vi "Run All Tests.vi"(8 "error in (no error)":errorcluster, 11 "Execution UI In":refnum<class "Execution UI V2.lvclass">) -> (0 "error out":errorcluster, 3 "Execution UI Out":refnum<class "Execution UI V2.lvclass">)   [LabVIEW 2020, in "Execution UI V2.lvclass"]
uses:
  Execution UI V2.lvclass
  Execution UI V2.lvclass/Execution UI V2.ctl
  Run/Runnable.lvclass
  Result Model/Result Model.lvclass
  TypeDefs/Execution State.ctl
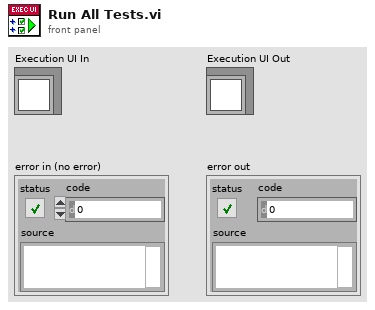
[diagram p1: front panel]
types:
  T1 = typedef "Execution UI V2.lvclass/Execution State.ctl" = enum16{"Idle", "Running"}
  T2 = typedef "Result.lvlib/Result.ctl" = cluster{"Name":string, "Message":string, "Description":string, "Status":T3, "Result Type":T4, "Execution Time":dbl}
  T3 = typedef "Result.lvlib/Status.ctl" = enum16{"", "Passed", "Failed", "Error", "Skipped", "Setup Error", "Broken", "Teardown Error"}
  T4 = typedef "Result.lvlib/Type.ctl" = enum16{"Method", "Case", "Suite", "Pass", "Fail", "Skip", "Pass if", "Fail if", "Pass if Error", "Fail if Error", "Pass if Equal", "Fail if Equal"}
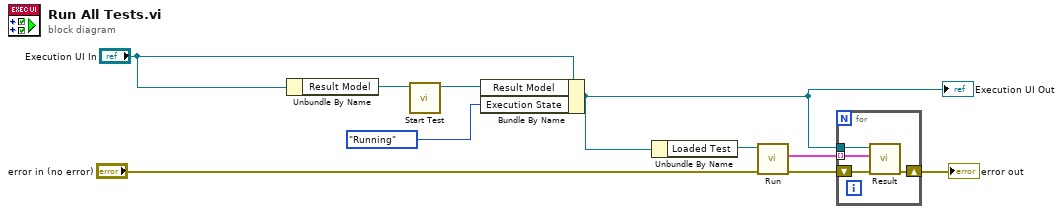
[diagram p0: block diagram]
diagram:
  n1 = Unbundle By Name("Execution UI In") -> ("Result Model"=w6:refnum<class "Result Model.lvclass">)
  n2 = call "Start Test.vi"("Result Model In"=w6) -> ("Result Model Out"=w5:refnum<class "Result Model.lvclass">)  [unwired: 10 in]
  n3 = Bundle By Name(cluster="Execution UI In", "Result Model"=w5, "Execution State"=Execution_State."Running") -> (w3:refnum<class "Execution UI V2.lvclass">)
  "Execution UI Out" <- w3
  n4 = Unbundle By Name(w3) -> ("Loaded Test"=w2:refnum<class "Runnable.lvclass">)
  n5 = call-dynamic "Run.vi"("error in (no error)"="error in (no error)", "Run in"=w2) -> ("error out"=w9:errorcluster, "Results"=w7:T2[])  [unwired: 8 in]
  n6 = for {
    tunnel: w3 -> [w14]
    tunnel: w7 -> [w11] mode=indexing
    shift-right: [w12] -> w8
    shift-left: w9 -> [w13]
    n7 = call-dynamic "Result.vi"("error in (no error)"=w13, "Result"=w11, "Execution UI V2 in"=w14) -> ("error out"=w12:errorcluster)  [unwired: 8 in]
  }
  "error out" <- w8
